vi "Test Save QOI (Path).vi"(8 "error in (no error)":errorcluster) -> (0 "error out":errorcluster, 3 "Pass?":bool)   [LabVIEW 2020]
uses:
  <vilib>/picture/picture.llb/imagedata.ctl
  G-Image/Image IO/Polymorphic VIs/Load Image (Path).vi
  G-Image/G-Image.lvlib
  G-Image/Image IO/Polymorphic VIs/Save QOI Image (Path).vi
panel:
  out "Array":cluster{string, "new picture":picture}[](array[cluster])
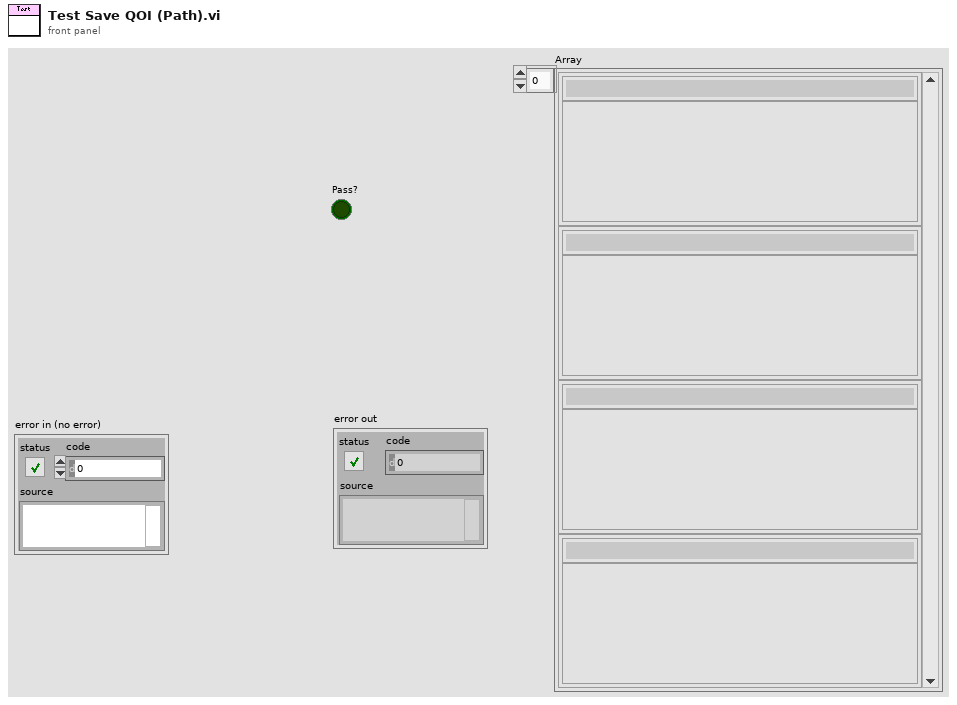
[diagram p1: front panel]
types:
  T1 = typedef "imagedata.ctl" = cluster{"image type":i32, "image depth":i32, "image":u8[], "mask":u8[], "colors":u32[], "Rectangle":cluster{"left":i16, "top":i16, "right":i16, "bottom":i16}}
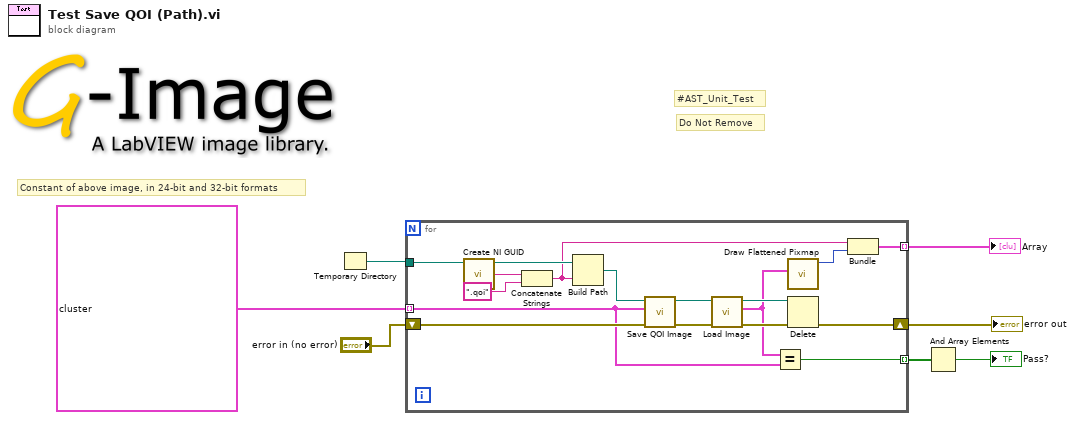
[diagram p0: block diagram]
diagram:
  # "Constant of above image, in 24-bit and 32-bit formats"
  # "Do Not Remove"
  # "#AST_Unit_Test"
  n1 = Temporary Directory() -> (w6:path)
  n2 = for {
    tunnel: w6 -> [w20]
    tunnel: T1[] [{"image type"=0, "image depth"=24, "image"=array[115500 elements], "mask"=[], "colors"=[], "Rectangle"={"left"=0, "top"=0, "right"=350, "bottom"=110}}, {"image type"=0, "image depth"=32, "image"=array[154000 elements], "mask"=array[4840 elements], "colors"=[], "Rectangle"={"left"=0, "top"=0, "right"=350, "bottom"=110}}] ("Array 2") -> [w16] mode=indexing
    shift-right: [w13] -> w4
    shift-left: "error in (no error)" -> [w23]
    tunnel: [w12] -> w3 mode=indexing
    tunnel: [w8] -> w5 mode=indexing
    n3 = call <vilib>:"Create NI GUID.vi"() -> ("NI GUID"=w21:string)
    n4 = Concatenate Strings(w21, ".qoi" ("string")) -> (w9:string)
    n5 = Build Path(base path=w20, name or relative path=w9) -> (appended path=w19:path)
    n6 = call-poly "Save QOI Image.vi"("error in (no error)"=w23, "Image"=w16, "Path In"=w19) -> ("error out"=w17:errorcluster, "Path Out"=w18:path)  [unwired: 7 in]
    n7 = call-poly "Load Image.vi"("error in (no error)"=w17, "Path In"=w18) -> ("error out"=w14:errorcluster, "Image"=w11:T1, "Path Out"=w15:path)  [unwired: 7 in]
    n8 = Equal?(x=w11, y=w16) -> (x = y?=w12:bool)
    n9 = call <vilib>:"Draw Flattened Pixmap.vi"("image data"=w11) -> ("new picture"=w10:picture)  [unwired: 8 in]
    n10 = Delete(path (use dialog)=w15, error in=w14) -> (error out=w13:errorcluster)  [unwired: 3 in, 2 out]
    n11 = Bundle(w9, "new picture"=w10) -> (w8:cluster{string, "new picture":picture})  [unwired: 1 in]
  }
  "error out" <- w4
  "Array" <- w5
  n12 = And Array Elements(Boolean array=w3) -> (logical AND=→"Pass?":bool)
